vi "Set Cooler.vi"(0 "Notifier Name":string, 7 "Cooler On?":bool, 11 "Error In":errorcluster) -> (4 "Notifier Name DUP":string, 15 "Error Out":errorcluster)   [LabVIEW 2020]
uses:
  Hardware Configuration/Hardware Configuration Controls/Company.ctl
  Hamamatsu/Orca Flash/Orca Flash Controls/Orca Flash Parameters.ctl
  Hamamatsu/Orca Flash/Orca Flash Controls/Orca Flash Parameter List.ctl
  Hamamatsu/Orca Flash/Orca Flash Controls/Orca Flash Actions.ctl
  <vilib>/vision/Image Controls.llb/IMAQ Image.ctl
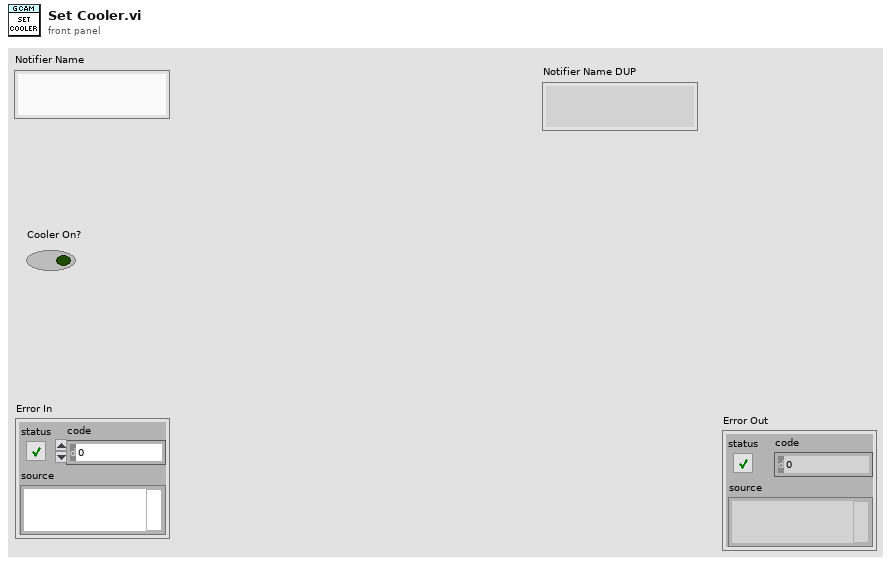
[diagram p1: front panel]
types:
  T1 = typedef "Company.ctl" = enum16{"AA Opto Electronic", "ASI", "Coherent", "Creset Optics", "CVI", "DAQmx", "Hamamatsu", "IDS", "Mad City Labs", "Marzhauser", "Measurement Computing", "MPB Com", "Olympus", "Photometrics", "PI", "Prior", "Thorlabs"}
  T2 = typedef "Orca Flash Actions.ctl" = enum16{"Idle", "Preview", "Record", "Record Settings", "Set Param", "Get Param", "Set ROI", "Get ROI", "Trigger Source", "Trigger Type", "Progessive Mode", "Area Mode", "Status", "Quit"}
  T3 = typedef "Orca Flash Parameters.ctl" = cluster{"Value":dbl, "Parameter":T4}
  T4 = typedef "Orca Flash Parameter List.ctl" = u32
  T5 = typedef "IMAQ Image.ctl" = refnum<image>
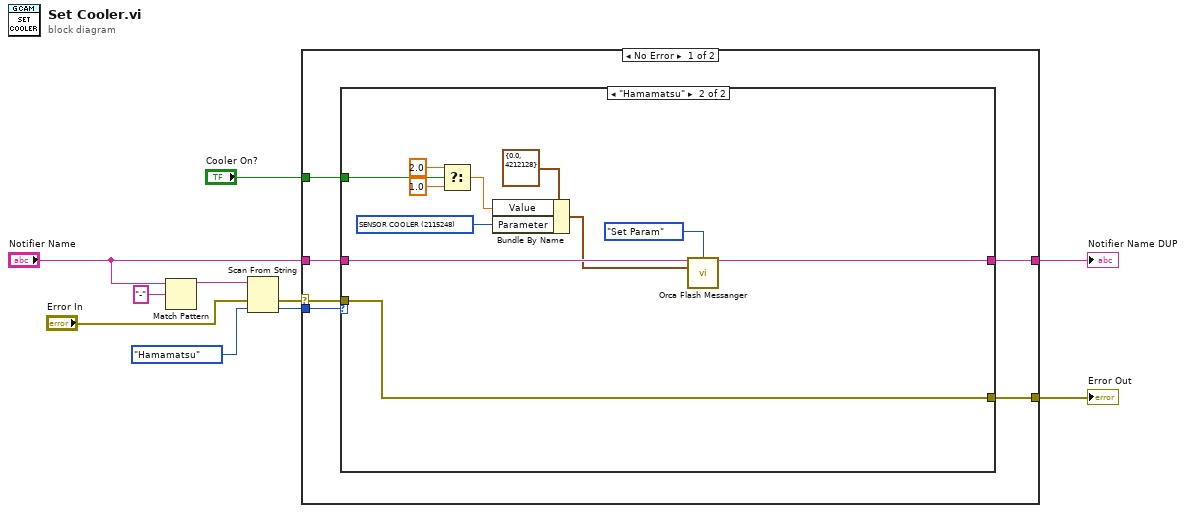
[diagram p0: block diagram]
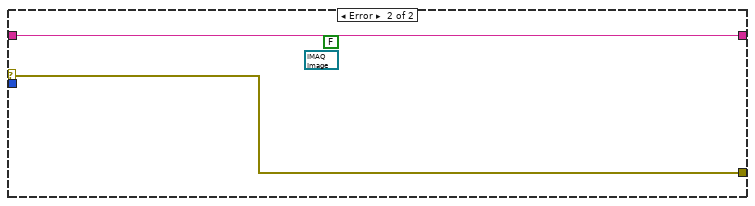
[diagram p3: hidden frame]
diagram:
  n1 = Match Pattern(string="Notifier Name", regular expression="-") -> (before substring=w8:string)  [unwired: 1 in, 3 out]
  n2 = Scan From String(input string=w8, error in="Error In", default 1=Company."Hamamatsu" ("Company")) -> (error out=w4:errorcluster, output 1=w7:T1)  [unwired: 2 in, 2 out]
  n3 = case shown="No Error" w4 {
    selector: w4 -> [w14 w30]
    tunnel: w7 -> [w16 _]
    tunnel: "Notifier Name" -> [w15 w31]
    tunnel: [w13 w31] -> w3
    tunnel: [w12 w30] -> w2
    tunnel: "Cooler On?" -> [w11 _]
    frame No Error {
      n4 = case shown="\"Hamamatsu\"" w16 {
        tunnel: w15 -> [w18 w29]
        tunnel: w14 -> [w17 w27]
        tunnel: [w18 w28] -> w13
        tunnel: [w17 w27] -> w12
        tunnel: w11 -> [_ w20]
        frame Default {
        }
        frame "Hamamatsu" {
          w26 = T4 2115248 items=["SENSOR MODE"=4212128, "READOUT SPEED"=4211872, "READOUT DIRECTION"=4211904, "TRIGGER GLOBAL EXPOSURE"=2049680, "TRIGGER DELAY"=1066480, "SYNC READOUT SYSTEM BLANK"=1066528, "SENSOR COOLER"=2115248, "SENSOR COOLER STATUS"=2115280, "EXPOSURE TIME"=2049184, "DEFECT CORRECT MODE"=4670368, "BINNING"=4215968, "INTERNAL LINE SPEED"=4226000, "INTERNAL LINE INTERVAL"=4226016, "IMAGE PIXEL TYPE"=4343296, "NUMBER OF OUTPUT TRIGGER CONNECTOR"=1852320, "OUTPUT TRIGGER SOURCE[0]"=1852576, "OUTPUT TRIGGER SOURCE[1]"=1852832, "OUTPUT TRIGGER SOURCE[2]"=1853088, "OUTPUT TRIGGER POLARITY[0]"=1852592, "OUTPUT TRIGGER POLARITY[1]"=1852848, "OUTPUT TRIGGER POLARITY[2]"=1853104, "OUTPUT TRIGGER ACTIVE[0]"=1852608, "OUTPUT TRIGGER ACTIVE[1]"=1852864, "OUTPUT TRIGGER ACTIVE[2]"=1853120, "OUTPUT TRIGGER DELAY[0]"=1852624, "OUTPUT TRIGGER DELAY[1]"=1852880, "OUTPUT TRIGGER DELAY[2]"=1853136, "OUTPUT TRIGGER PERIOD[0]"=1852640, "OUTPUT TRIGGER PERIOD[1]"=1852896, "OUTPUT TRIGGER PERIOD[2]"=1853152, "OUTPUT TRIGGER KIND[0]"=1852656, "OUTPUT TRIGGER KIND[1]"=1852912, "OUTPUT TRIGGER KIND[2]"=1853168, "OUTPUT TRIGGER PRE HSYNC COUNT"=1852704] ("Parameter")
          n5 = Select(t=2.0, s=w20, f=1.0) -> (s? t:f=w21:dbl)
          n6 = Bundle By Name(cluster=T3 {"Value"=0.0, "Parameter"=4212128} ("sCMOS Parameter"), "Value"=w21, "Parameter"=w26) -> (w24:T3)
          n7 = call "Orca Flash Messanger.vi"("Notifier Name"=w29, "Camera Actions"=Orca_Flash_Actions."Set Param", "sCMOS Parameter"=w24) -> ("Notifier Name Dup"=w28:string)  [unwired: 8 in, 4 out]
        }
      }
    }
    frame Error {
      (unwired) T5 refnum ("Image Ref")
      (unwired) FALSE ("Running?")
    }
  }
  "Error Out" <- w2
  "Notifier Name DUP" <- w3
